vi "Varient_Creator.vi"(8 "error in (no error)":errorcluster) -> (0 "error out":errorcluster)   [LabVIEW 2017]
uses:
  <vilib>/Utility/file.llb/Read Delimited Spreadsheet (string).vi
  <vilib>/Utility/file.llb/Write Delimited Spreadsheet (string).vi
  <vilib>/Utility/config.llb/NI_LVConfig.lvlib
  557cc533-a4ba-4953-a7b5-ba01b5e60265.vi
panel:
  in  "Varient Details":string[][](table)
  in  "Test Resistor":string(combo)
  in  "Magnetic Asyl":string(combo)
  in  "Kinematic Asyl":string(combo)
  in  "CBCT Group":string(combo)
  in  "PMR":string(combo)
  in  "Hausing No":string(combo)
  in  "Delete Button":bool
  in  "Save Button":bool
  in  "Sr  No":u16=1 min=1 max=100 step=1
  in  "HOME":bool
  in  "UPDATE TABLE":bool
  in  "FG CAT No":string(combo)
  # "Varient Creater"
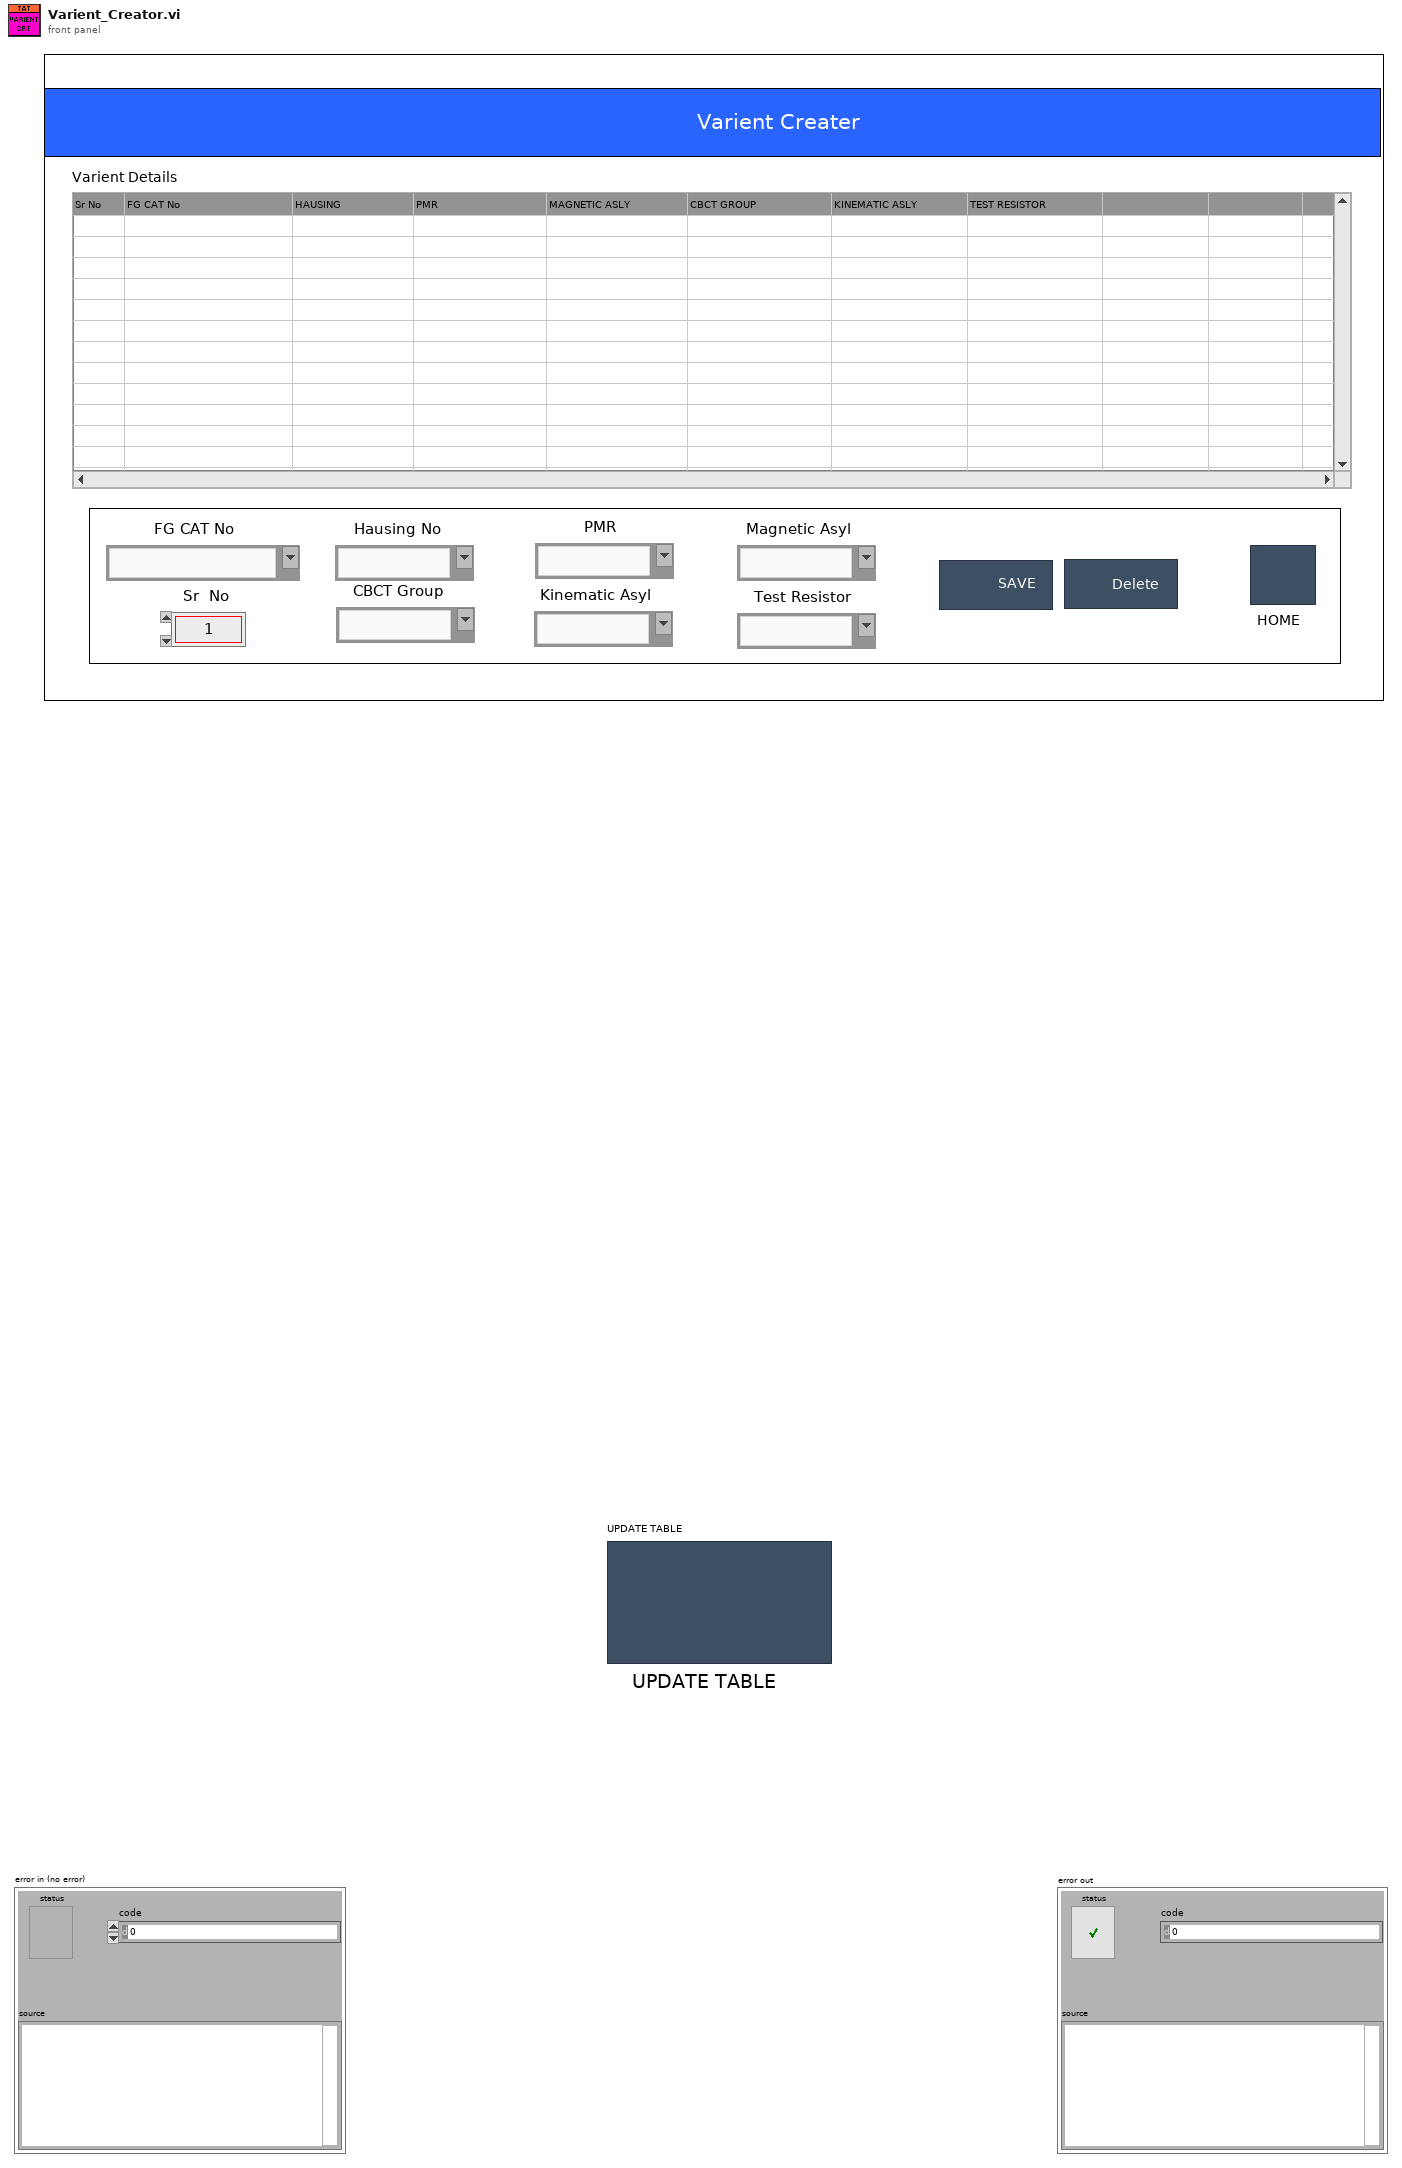
[diagram p1: front panel]
types:
  T1 = enum32{"invalid app kind", "Development System", "Run Time System", "Student Edition", "Embedded LabVIEW", "Evaluation", "Custom"}
  T2 = typedef "NI_LVConfig.lvlib/Config Data RefNum.ctl" = refnum<k1>
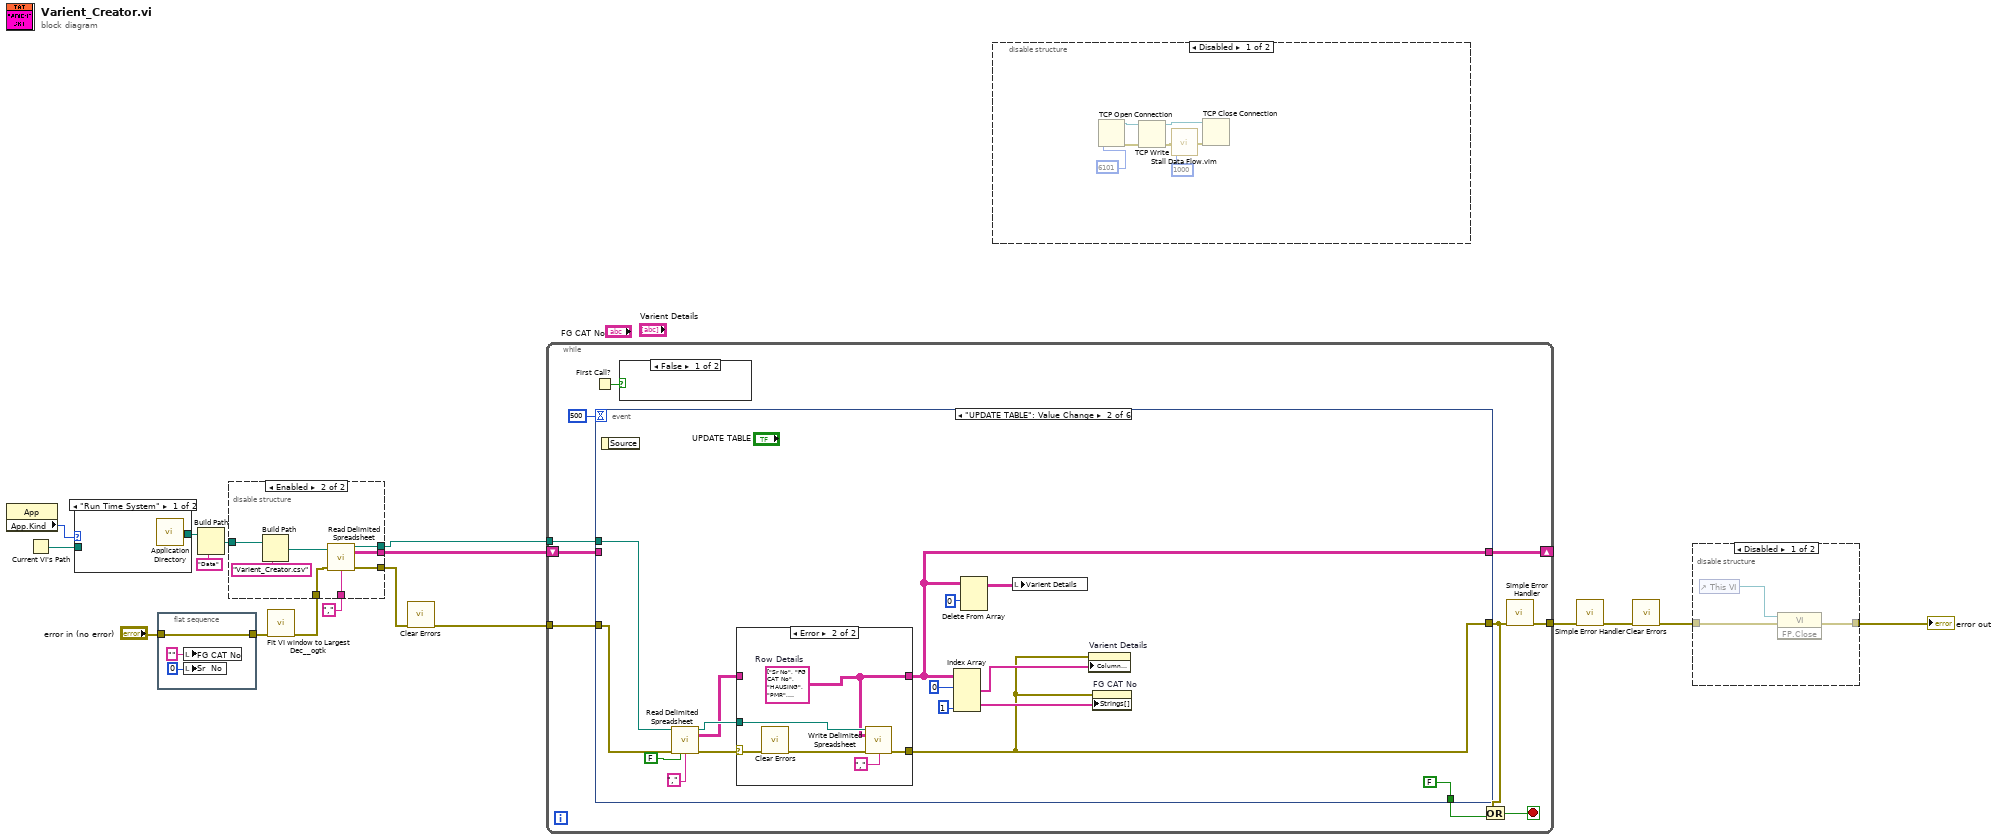
[diagram p0: block diagram]
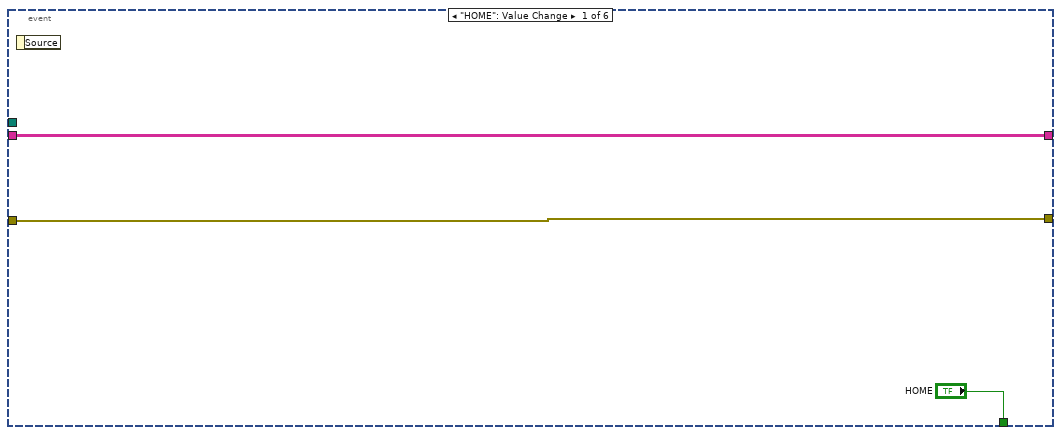
[diagram p3: hidden frame]
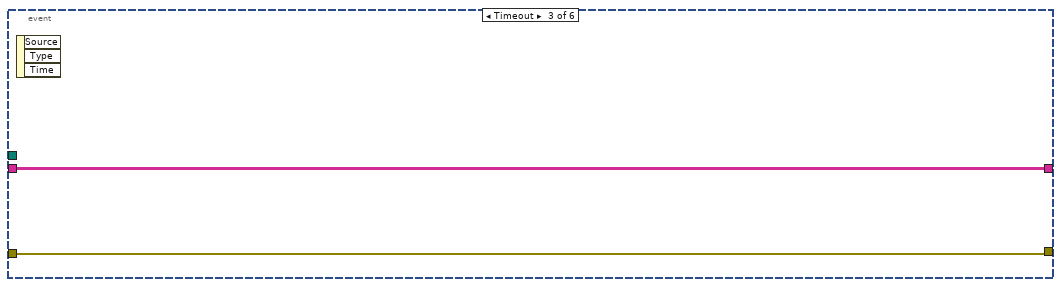
[diagram p5: hidden frame]
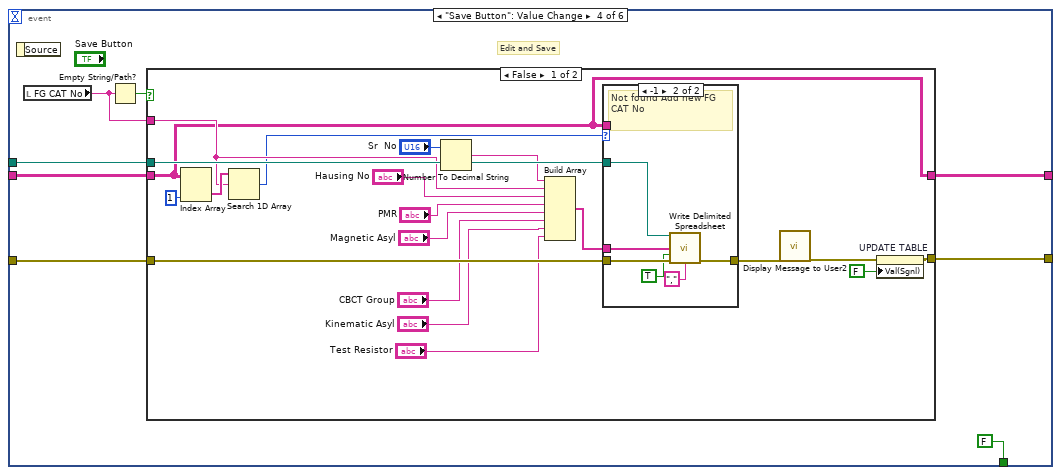
[diagram p6: hidden frame]
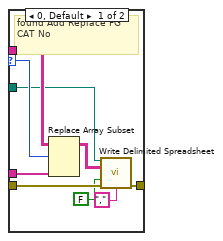
[diagram p7: hidden frame]
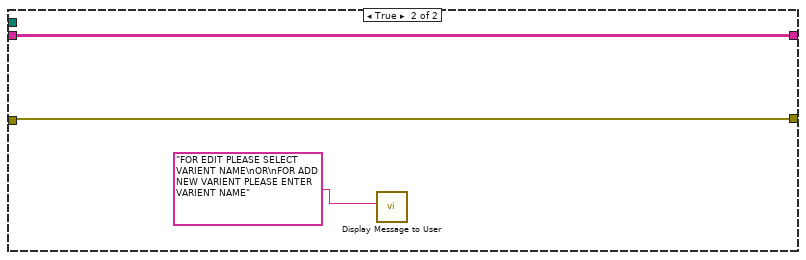
[diagram p8: hidden frame]
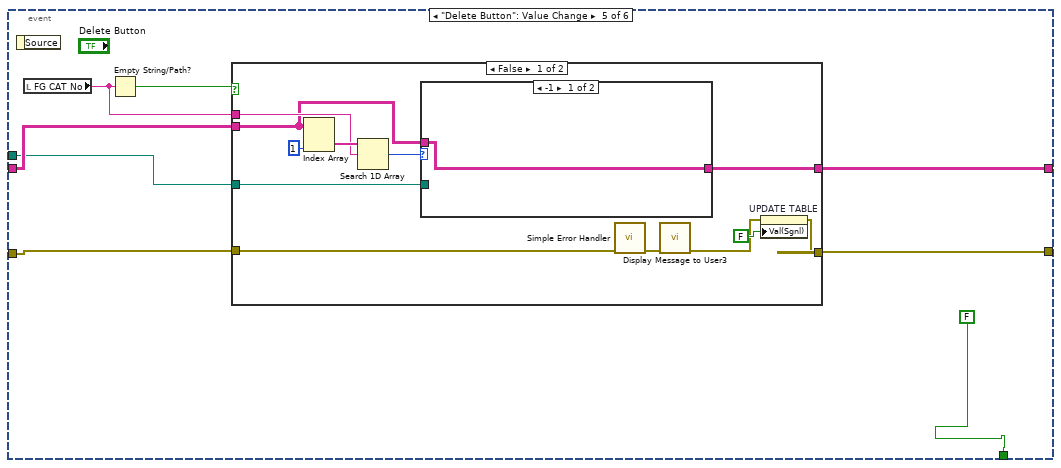
[diagram p9: hidden frame]
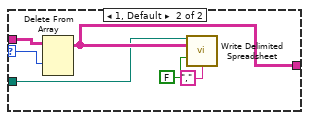
[diagram p10: hidden frame]
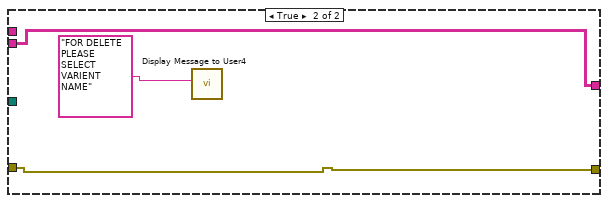
[diagram p11: hidden frame]
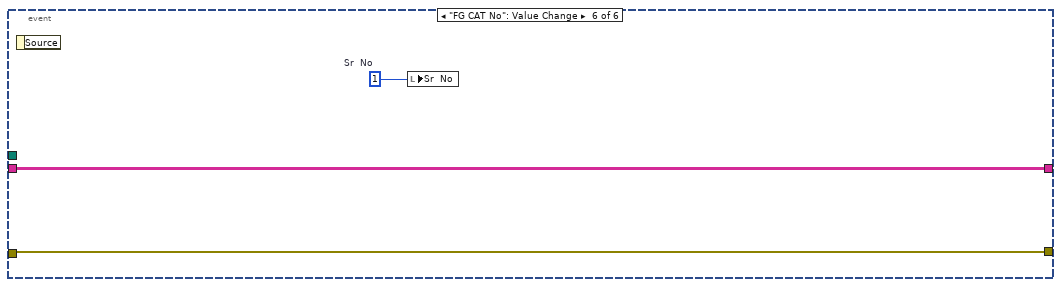
[diagram p12: hidden frame]
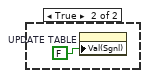
[diagram p13: hidden frame]
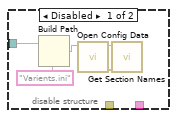
[diagram p15: hidden frame]
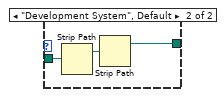
[diagram p16: hidden frame]
diagram:
  n1 = property class="App"() -> ("App.Kind"=w10:T1)  [unwired: 2 in, 2 out]
  n2 = Current VI's Path() -> (path=w11:path)
  n3 = case shown="\"Run Time System\"" w10 {
    tunnel: w11 -> [_ w20]
    tunnel: [w18 w19] -> w7
    frame "Run Time System" {
      n4 = call <vilib>:"Application Directory.vi"() -> ("Application Directory"=w18:path)
    }
    frame "Development System", Default {
      n5 = Strip Path(path=w20) -> (stripped path=w21:path)  [unwired: 1 out]
      n6 = Strip Path(path=w21) -> (stripped path=w19:path)  [unwired: 1 out]
    }
  }
  n7 = flat-sequence {
    tunnel: [w24] -> w12
    tunnel: "error in (no error)" -> [w24]
    frame #0 {
      n8 = local write "FG CAT No"("" ("PART NUMBER")) -> ()
      n9 = local write "Sr  No"(u16 0 ("BATCH SIZE")) -> ()
    }
  }
  n10 = Build Path(base path=w7, name or relative path="Data") -> (appended path=w8:path)
  n11 = call <userlib>:"Fit VI window to Largest Dec__ogtk.vi"("error in (no error)"=w12) -> ("error out"=w4:errorcluster)  [unwired: 5 in, 1 out]
  n12 = disable-structure shown="Enabled" {
    disable-tunnel: w8 -> [w25 w36]
    disable-tunnel: w4 -> [_ w34]
    disable-tunnel: [_ w33] -> w6
    disable-tunnel: [_ w32] -> w5
    disable-tunnel: [_ w31] -> w3
    disable-tunnel: "," -> [_ w30]
    frame Disabled {
      n13 = Build Path(base path=w25, name or relative path="Varients.ini") -> (appended path=w29:path)
      n14 = call <vilib>:"Open Config Data.vi"("configuration file path"=w29) -> ("error out"=w26:errorcluster, "refnum"=w27:T2)  [unwired: 8 in, 1 out]
      n15 = call <vilib>:"Get Section Names.vi"("error in (no error)"=w26, "refnum"=w27) -> ()  [unwired: 7 in, 3 out]
    }
    frame Enabled {
      n16 = Build Path(base path=w36, name or relative path="Varient_Creator.csv") -> (appended path=w35:path)
      n17 = call-poly <vilib>:"Read Delimited Spreadsheet.vi"("file path (dialog if empty)"=w35, "error in (no error)"=w34, "delimiter (\\t)"=w30) -> ("new file path (Not A Path if cancelled)"=w32:path, "all rows"=w33:string[][], "error out"=w31:errorcluster)  [unwired: 7 in, 3 out]
    }
  }
  n18 = call <vilib>:"Clear Errors.vi"("error in (no error)"=w3) -> ("error out"=w2:errorcluster)  [unwired: 5 in, 1 out]
  n19 = while {
    tunnel: [w41] -> w14
    tunnel: w2 -> [w44]
    tunnel: w5 -> [w43]
    shift-right: [w40] -> _
    shift-left: w6 -> [w38]
    stop <- w46 stop-if-true
    n20 = First Call?() -> (First Call?: T/F=w45:bool)
    n21 = event shown="[1] \"UPDATE TABLE\": Value Change" {
      selector: _ -> [_ _ _ _ _ _]
      dyn-events: _ -> [_ _ _ _ _ _]
      timeout: 500 -> [_ _ _ _ _ _]
      tunnel: ["HOME" FALSE ("stop") _ FALSE ("stop") FALSE ("stop") _] -> w47
      tunnel: [w49 w54 w75 w82 w127 w153] -> w42
      tunnel: w44 -> [w49 w65 w75 w80 w126 w153]
      tunnel: w38 -> [w48 _ w76 w79 w125 w154]
      tunnel: w43 -> [_ w64 _ w78 w123 _]
      tunnel: [w48 w51 w76 w77 w124 w154] -> w40
      event "HOME": Value Change {
        n22 = event-data() -> ()  [unwired: 1 in, 1 out]
      }
      event "UPDATE TABLE": Value Change {
        n23 = event-data() -> ()  [unwired: 1 in, 1 out]
        n24 = call-poly <vilib>:"Read Delimited Spreadsheet.vi"("file path (dialog if empty)"=w64, "error in (no error)"=w65, "transpose? (F)"=FALSE, "delimiter (\\t)"=",") -> ("new file path (Not A Path if cancelled)"=w60:path, "all rows"=w59:string[][], "error out"=w61:errorcluster)  [unwired: 6 in, 3 out]
        n25 = case shown="Error" w61 {
          selector: w61 -> [w68 w74]
          tunnel: [w68 w72] -> w54
          tunnel: w60 -> [_ w71]
          tunnel: [w67 w69] -> w51
          tunnel: w59 -> [w67 _]
          frame No Error {
          }
          frame Error {
            w69 = string[][] [["Sr No", "FG CAT No", "HAUSING", "PMR", "MAGNETIC ASLY", "CBCT GROUP", "KINEMATIC ASLY", "TEST RESISTOR"]]  # Row Details
            n26 = call <vilib>:"Clear Errors.vi"("error in (no error)"=w74) -> ("error out"=w73:errorcluster)  [unwired: 5 in, 1 out]
            n27 = call-poly <vilib>:"Write Delimited Spreadsheet.vi"("file path (dialog if empty)"=w71, "2D data"=w69, "error in (no error)"=w73, "delimiter (\\t)"=",") -> ("error out"=w72:errorcluster)  [unwired: 10 in, 1 out]
          }
        }
        n28 = Index Array(array=w51, index (row) #1=0, index (col) #2=1) -> (element #1=w55:string[], element #2=w57:string[])  [unwired: 2 in]
        n29 = Delete From Array(array=w51, index (row)=0) -> (array with subset deleted=w53:string[][])  [unwired: 2 in, 1 out]
        n30 = local write "Varient Details"(w53) -> ()
        n31 = property on="Varient Details" class="Tbl (strict)"(error in=w54, "Column Headers[]"=w55) -> ()  [unwired: 1 in, 2 out]
        n32 = property on="FG CAT No" class="CmbBox"(error in=w54, "Strings[]"=w57) -> ()  [unwired: 1 in, 2 out]
      }
      event Timeout {
        n33 = event-data() -> ()  [unwired: 1 in, 3 out]
      }
      event "Save Button": Value Change {
        # "Edit and Save"
        n34 = event-data() -> ()  [unwired: 1 in, 1 out]
        n35 = local read "FG CAT No"() -> (w83:string)
        n36 = Empty String/Path?(string/path=w83) -> (empty?=w81:bool)
        n37 = case shown="False" w81 {
          tunnel: [w103 w121] -> w82
          tunnel: w83 -> [w96 _]
          tunnel: w80 -> [w100 w121]
          tunnel: w79 -> [w90 w120]
          tunnel: w78 -> [w101 _]
          tunnel: [w90 w120] -> w77
          frame False {
            n38 = Index Array(array=w90, index (col)=1) -> (element=w97:string[])  [unwired: 1 in]
            n39 = Search 1D Array(1D array=w97, element=w96) -> (index of element=w91:i32)  [unwired: 1 in]
            n40 = Number To Decimal String(number="Sr  No") -> (decimal integer string=w94:string)  [unwired: 1 in]
            n41 = Build Array(w94, w96, "Hausing No", "PMR", "Magnetic Asyl", "CBCT Group", "Kinematic Asyl", "Test Resistor") -> (w92:string[])
            n42 = case shown="-1" w91 {
              selector: w91 -> [w109 _]
              tunnel: w101 -> [w107 w119]
              tunnel: w100 -> [w112 w118]
              tunnel: [w113 w117] -> w99
              tunnel: w92 -> [w110 w115]
              tunnel: w90 -> [w111 _]
              frame 0, Default {
                # "found Add Replace FG CAT No"
                n43 = Replace Array Subset(array=w111, new element=w110, index (row)=w109) -> (w108:string[][])  [unwired: 1 in]
                n44 = call-poly <vilib>:"Write Delimited Spreadsheet.vi"("file path (dialog if empty)"=w107, "2D data"=w108, "append to file? (new file:F)"=FALSE, "error in (no error)"=w112, "delimiter (\\t)"=",") -> ("error out"=w113:errorcluster)  [unwired: 9 in, 1 out]
              }
              frame -1 {
                # "Not found Add new FG CAT No"
                n45 = call-poly <vilib>:"Write Delimited Spreadsheet.vi"("file path (dialog if empty)"=w119, "1D data"=w115, "append to file? (new file:F)"=TRUE, "error in (no error)"=w118, "delimiter (\\t)"=",") -> ("error out"=w117:errorcluster)  [unwired: 9 in, 1 out]
              }
            }
            n46 = call "Display Message to User2"("error in (no error)"=w99) -> ("error out"=w102:errorcluster)  [unwired: 9 in, 1 out]
            n47 = property on="UPDATE TABLE" class="Bool (strict)"(error in=w102, "Val(Sgnl)"=FALSE) -> (error out=w103:errorcluster)  [unwired: 1 in, 1 out]
          }
          frame True {
            n48 = call "Display Message to User"("Message"="FOR EDIT PLEASE SELECT VARIENT NAME\nOR\nFOR ADD NEW VARIENT PLEASE ENTER VARIENT NAME") -> ()  [unwired: 9 in, 2 out]
          }
        }
      }
      event "Delete Button": Value Change {
        n49 = event-data() -> ()  [unwired: 1 in, 1 out]
        n50 = local read "FG CAT No"() -> (w129:string)
        n51 = Empty String/Path?(string/path=w129) -> (empty?=w128:bool)
        n52 = case shown="False" w128 {
          tunnel: [w141 w151] -> w127
          tunnel: w129 -> [w135 _]
          tunnel: w126 -> [w138 w151]
          tunnel: w125 -> [w133 w150]
          tunnel: [w132 w150] -> w124
          tunnel: w123 -> [w131 _]
          frame False {
            n53 = Index Array(array=w133, index (col)=1) -> (element=w136:string[])  [unwired: 1 in]
            n54 = Search 1D Array(1D array=w136, element=w135) -> (index of element=w134:i32)  [unwired: 1 in]
            n55 = case shown="-1" w134 {
              selector: w134 -> [_ w148]
              tunnel: w133 -> [w143 w149]
              tunnel: [w143 w145] -> w132
              tunnel: w131 -> [_ w144]
              frame -1 {
              }
              frame 1, Default {
                n56 = Delete From Array(array=w149, index (row)=w148) -> (array with subset deleted=w145:string[][])  [unwired: 2 in, 1 out]
                n57 = call-poly <vilib>:"Write Delimited Spreadsheet.vi"("file path (dialog if empty)"=w144, "2D data"=w145, "append to file? (new file:F)"=FALSE, "delimiter (\\t)"=",") -> ()  [unwired: 10 in, 2 out]
              }
            }
            n58 = call <vilib>:"Simple Error Handler.vi"("error in (no error)"=w138) -> ("error out"=w140:errorcluster)  [unwired: 4 in, 4 out]
            n59 = call "Display Message to User3"("error in (no error)"=w140) -> ("error out"=w139:errorcluster)  [unwired: 9 in, 1 out]
            n60 = property on="UPDATE TABLE" class="Bool (strict)"(error in=w139, "Val(Sgnl)"=FALSE) -> (error out=w141:errorcluster)  [unwired: 1 in, 1 out]
          }
          frame True {
            n61 = call "Display Message to User4"("Message"="FOR DELETE PLEASE SELECT VARIENT NAME") -> ()  [unwired: 9 in, 2 out]
          }
        }
      }
      event "FG CAT No": Value Change {
        w155 = u16 1  # Sr  No
        n62 = event-data() -> ()  [unwired: 1 in, 1 out]
        n63 = local write "Sr  No"(w155) -> ()
      }
    }
    n64 = case shown="False" w45 {
      frame False {
      }
      frame True {
        n65 = property on="UPDATE TABLE" class="Bool (strict)"("Val(Sgnl)"=FALSE) -> ()  [unwired: 2 in, 2 out]
      }
    }
    n66 = Or(x=w42, y=w47) -> (x .or. y?=w46:bool)
    n67 = call <vilib>:"Simple Error Handler.vi"("error in (no error)"=w42) -> ("error out"=w41:errorcluster)  [unwired: 4 in, 4 out]
  }
  n68 = disable-structure shown="Disabled" {
    frame Disabled {
      n69 = TCP Open Connection(remote port or service name=u16 6101) -> (connection ID=w162:refnum<k5>, error out=w161:errorcluster)  [unwired: 4 in]
      n70 = TCP Write(connection ID=w162, error in (no error)=w161) -> (connection ID out=w164:refnum<k5>, error out=w160:errorcluster)  [unwired: 2 in, 1 out]
      n71 = call "Stall Data Flow.vim"("value in"=w160, "milliseconds to wait"=u32 1000) -> ("value out"=w163:errorcluster)  [unwired: 1 out]
      n72 = TCP Close Connection(connection ID=w164, error in (no error)=w163) -> (error out=w157:errorcluster)  [unwired: 1 in, 1 out]
    }
    frame Enabled {
    }
  }
  n73 = call <vilib>:"Simple Error Handler.vi"("error in (no error)"=w14) -> ("error out"=w17:errorcluster)  [unwired: 4 in, 4 out]
  n74 = call <vilib>:"Clear Errors.vi"("error in (no error)"=w17) -> ("error out"=w16:errorcluster)  [unwired: 5 in, 1 out]
  n75 = disable-structure shown="Disabled" {
    disable-tunnel: w16 -> [w167 w168]
    disable-tunnel: [w166 w168] -> w15
    frame Disabled {
      n76 = control-ref of="This VI"() -> (w165:refnum<vi>)
      n77 = invoke class="VI" method="FP.Close"(reference=w165, error in=w167) -> (error out=w166:errorcluster)  [unwired: 1 in, 2 out]
    }
    frame Enabled {
    }
  }
  "error out" <- w15
